vi "OnResize2.vi"(0 "XRef":T20, 1 "Bounds":T18, 2 "Mouse Mods":T16, 3 "State In":T1={"Worker Library Path"=path "", "Block Label"="", "Types"=[], "Selections"=[], "Icon"={"image type"=0, "image depth"=0, "image"=[], "mask"=[], "colors"=[], "Rectangle"={"left"=0, "top"=0, "right"=0, "bottom"=0}}, "Errors"={"Terminals"=[], "Generate"={"status"=FALSE, "code"=0, "source"=""}, "General"={"status"=FALSE, "code"=0, "source"=""}}, "Calculated Sizes"={"Block Width"=0, "Block Height"=0, "Half Width"=0, "Icon Top"=0, "Icon Bottom"=0, "Label Width"=0, "Half Label"=0, "Label Top"=0, "Text Width"=0, "Half Text"=0, "Text Height"=0, "Label Height"=0, "Expanded Width"=0, "Label Bottom"=0, "Expanded Top"=0, "Expanded Bottom"=0, "Expanded Height"=0, "Min Height"=0, "Max Height"=0}, "Special Terminal Indices"={"Action"=-1, "Init"=-1, "Tag"=-1, "State in"=-1, "State out"=-1, "Error"=-1, "Control"=-1}, "Terminals"=[], "First Gen?"=FALSE}) -> (14 "Reply":T14, 15 "Fatal Error Out":T13, 16 "State Out":T1={"Worker Library Path"=path "", "Block Label"="", "Types"=[], "Selections"=[], "Icon"={"image type"=0, "image depth"=0, "image"=[], "mask"=[], "colors"=[], "Rectangle"={"left"=0, "top"=0, "right"=0, "bottom"=0}}, "Errors"={"Terminals"=[], "Generate"={"status"=FALSE, "code"=0, "source"=""}, "General"={"status"=FALSE, "code"=0, "source"=""}}, "Calculated Sizes"={"Block Width"=0, "Block Height"=0, "Half Width"=0, "Icon Top"=0, "Icon Bottom"=0, "Label Width"=0, "Half Label"=0, "Label Top"=0, "Text Width"=0, "Half Text"=0, "Text Height"=0, "Label Height"=0, "Expanded Width"=0, "Label Bottom"=0, "Expanded Top"=0, "Expanded Bottom"=0, "Expanded Height"=0, "Min Height"=0, "Max Height"=0}, "Special Terminal Indices"={"Action"=-1, "Init"=-1, "Tag"=-1, "State in"=-1, "State out"=-1, "Error"=-1, "Control"=-1}, "Terminals"=[], "First Gen?"=FALSE})   [LabVIEW 2022 SP3, in "Flex Block.xnode"]
uses:
  Flex Block.xnode
  <vilib>/XNodeSupport/XNodeXNodeRef.ctl
  <vilib>/XNodeSupport/XNodeRect32.ctl
  <vilib>/XNodeSupport/XNodeInt.ctl
  <vilib>/XNodeSupport/XNodeMouseMods.ctl
  <vilib>/XNodeSupport/XNodeBool.ctl
  State.ctl
  FlexBlocks Support/Type Descriptor.ctl
  FlexBlocks Support/Terminal Direction.ctl
  FlexBlocks Support/Value Mode.ctl
  FlexBlocks Support/Special Terminal.ctl
  <vilib>/picture/picture.llb/imagedata.ctl
  FlexBlocks Support/XNode Errors.ctl
  FlexBlocks Support/Calculated Sizes.ctl
  FlexBlocks Support/Special Terminal Indices.ctl
  FlexBlocks Support/Terminal Status.ctl
  FlexBlocks Support/Terminal State.ctl
  FlexBlocks Support/Terminal Draw Style.ctl
  <vilib>/XNodeSupport/XNodeStringArray.ctl
  <vilib>/XNodeSupport/XNodeString.ctl
  <vilib>/XNodeSupport/XNodeErrorCluster.ctl
  3ea49023-45ad-42f1-9e97-9f20a21117f8.vi
  FlexBlocks Support/_Add Ability Log.vi
  <vilib>/XNodeSupport/NI_XNodeSupport.lvlib
  FlexBlocks Support/FlexBlocks Support.lvlib
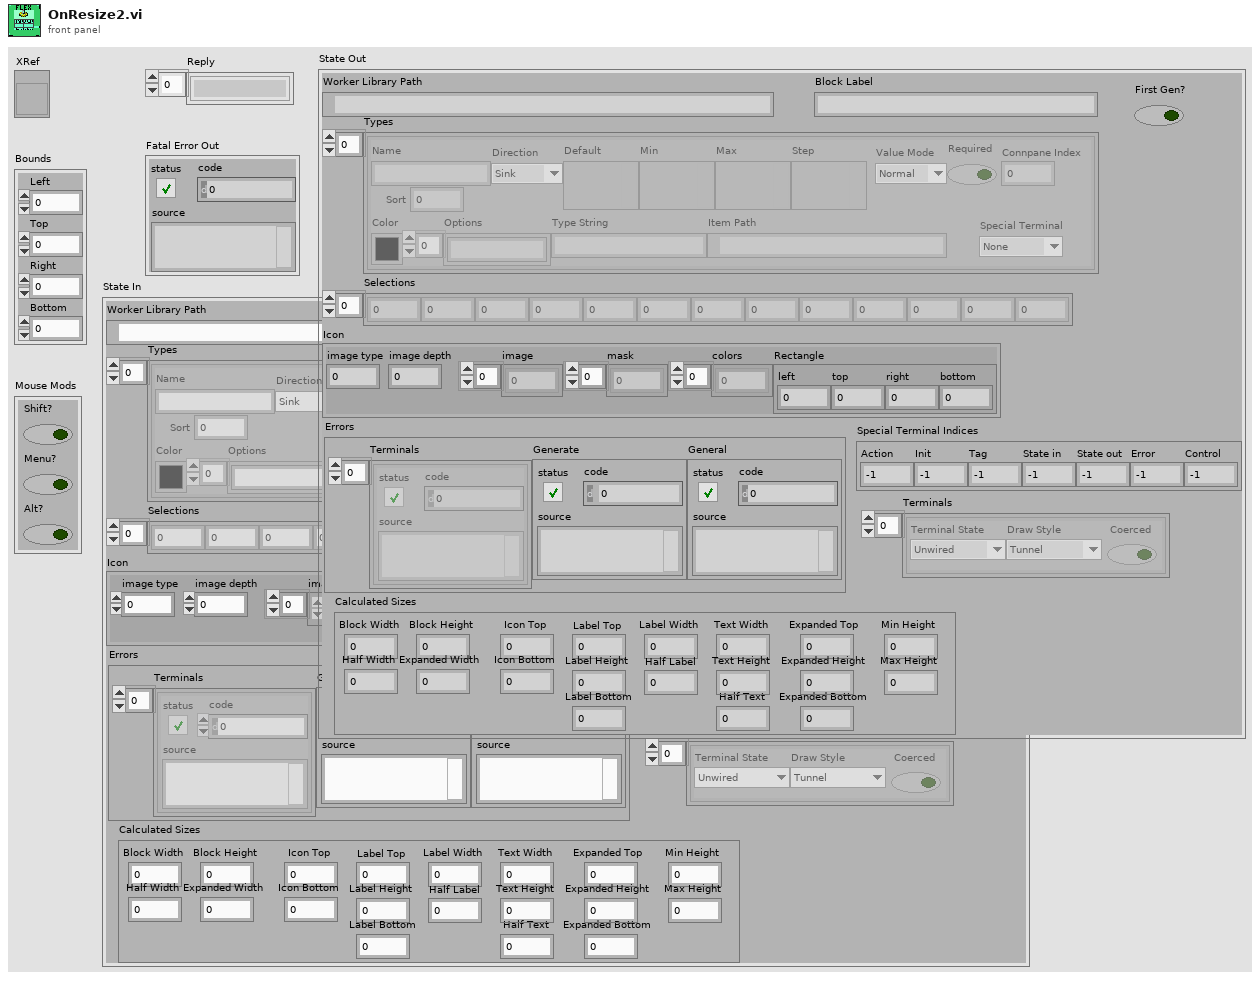
[diagram p1: front panel]
types:
  T1 = typedef "Flex Block.xnode/State.ctl" = cluster{"Worker Library Path":path, "Block Label":string, "Types":T2[], "Selections":i32[], "Icon":T6, "Errors":T7, "Calculated Sizes":T8, "Special Terminal Indices":T9, "Terminals":T10[], "First Gen?":bool}
  T2 = typedef "FlexBlocks Support.lvlib/Type Descriptor.ctl" = cluster{"Name":string, "Direction":T3, "Default":variant, "Min":variant, "Max":variant, "Step":variant, "Value Mode":T4, "Color":u32, "Options":string[], "Type String":string, "Item Path":path, "Required":bool, "Connpane Index":i32, "Special Terminal":T5, "Sort":i32}
  T3 = typedef "FlexBlocks Support.lvlib/Terminal Direction.ctl" = enum16{"Sink", "Source"}
  T4 = typedef "FlexBlocks Support.lvlib/Value Mode.ctl" = enum16{"Normal", "Range", "Select"}
  T5 = typedef "FlexBlocks Support.lvlib/Special Terminal.ctl" = enum16{"None", "Action", "Init", "Tag", "State in", "State out", "Error", "Control"}
  T6 = typedef "imagedata.ctl" = cluster{"image type":i32, "image depth":i32, "image":u8[], "mask":u8[], "colors":u32[], "Rectangle":cluster{"left":i16, "top":i16, "right":i16, "bottom":i16}}
  T7 = typedef "FlexBlocks Support.lvlib/XNode Errors.ctl" = cluster{"Terminals":errorcluster[], "Generate":errorcluster, "General":errorcluster}
  T8 = typedef "FlexBlocks Support.lvlib/Calculated Sizes.ctl" = cluster{"Block Width":i32, "Block Height":i32, "Half Width":i32, "Icon Top":i32, "Icon Bottom":i32, "Label Width":i32, "Half Label":i32, "Label Top":i32, "Text Width":i32, "Half Text":i32, "Text Height":i32, "Label Height":i32, "Expanded Width":i32, "Label Bottom":i32, "Expanded Top":i32, "Expanded Bottom":i32, "Expanded Height":i32, "Min Height":i32, "Max Height":i32}
  T9 = typedef "FlexBlocks Support.lvlib/Special Terminal Indices.ctl" = cluster{"Action":i32, "Init":i32, "Tag":i32, "State in":i32, "State out":i32, "Error":i32, "Control":i32}
  T10 = typedef "FlexBlocks Support.lvlib/Terminal Status.ctl" = cluster{"Terminal State":T11, "Draw Style":T12, "Coerced":bool}
  T11 = typedef "FlexBlocks Support.lvlib/Terminal State.ctl" = enum16{"Unwired", "BadType", "BadRef", "Channel", "Value", "Control Ref"}
  T12 = typedef "FlexBlocks Support.lvlib/Terminal Draw Style.ctl" = enum16{"Tunnel", "BadType", "BadRef", "Channel", "Value", "Control Ref"}
  T13 = typedef "NI_XNodeSupport.lvlib/XNodeErrorCluster.ctl" = errorcluster
  T14 = typedef "NI_XNodeSupport.lvlib/XNodeStringArray.ctl" = T15[]
  T15 = typedef "NI_XNodeSupport.lvlib/XNodeString.ctl" = string
  T16 = typedef "NI_XNodeSupport.lvlib/XNodeMouseMods.ctl" = cluster{"Shift?":T17, "Menu?":T17, "Alt?":T17}
  T17 = typedef "NI_XNodeSupport.lvlib/XNodeBool.ctl" = bool
  T18 = typedef "NI_XNodeSupport.lvlib/XNodeRect32.ctl" = cluster{"Left":T19, "Top":T19, "Right":T19, "Bottom":T19}
  T19 = typedef "NI_XNodeSupport.lvlib/XNodeInt.ctl" = i32
  T20 = typedef "NI_XNodeSupport.lvlib/XNodeXNodeRef.ctl" = refnum<vi>
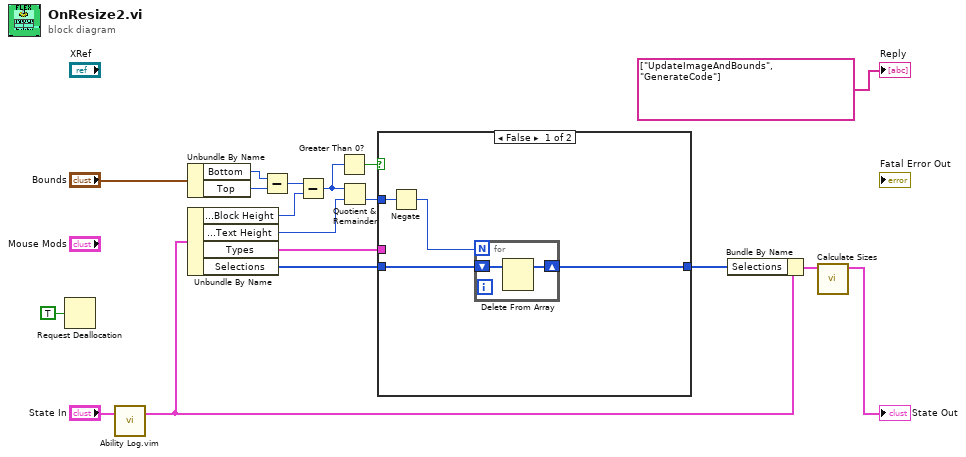
[diagram p0: block diagram]
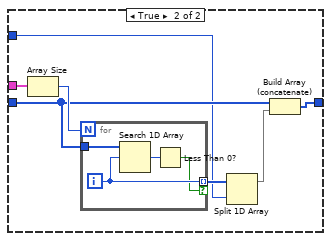
[diagram p2: hidden frame]
diagram:
  n1 = Request Deallocation(TRUE ("flag")) -> ()
  n2 = call "Ability Log.vim"("Wire in"="State In") -> ("Wire out"=w1:T1)  [unwired: 6 in]
  n3 = Unbundle By Name("Bounds") -> ("Bottom"=w15:T19, "Top"=w16:T19)
  n4 = Unbundle By Name(w1) -> ("Calculated Sizes.Block Height"=w13:i32, "Calculated Sizes.Text Height"=w3:i32, "Types"=w12:T2[], "Selections"=w11:i32[])
  n5 = Subtract(x=w15, y=w16) -> (x-y=w14:T19)
  n6 = Subtract(x=w14, y=w13) -> (x-y=w4:T19)
  n7 = Greater Than 0?(x=w4) -> (x > 0?=w8:bool)
  n8 = Quotient & Remainder(x=w4, y=w3) -> (floor(x/y)=w5:T19)  [unwired: 1 out]
  n9 = case shown="False" w8 {
    tunnel: w12 -> [_ w31]
    tunnel: w11 -> [w22 w28]
    tunnel: [w21 w26] -> w10
    tunnel: w5 -> [w20 w25]
    frame False {
      n10 = Negate(x=w20) -> (-x=w19:T19)
      n11 = for {
        N: w19 -> [_]
        shift-right: [w23] -> w21
        shift-left: w22 -> [w24]
        n12 = Delete From Array(array=w24) -> (array with subset deleted=w23:i32[])  [unwired: 2 in, 1 out]
      }
    }
    frame True {
      n13 = Array Size(array=w31) -> (size(s)=w30:i32)
      n14 = for {
        N: w30 -> [_]
        tunnel: w28 -> [w35]
        tunnel: [w33] -> w29 mode=indexing if=w32
        i -> [w33]
        n15 = Search 1D Array(1D array=w35, element=w33) -> (index of element=w34:i32)  [unwired: 1 in]
        n16 = Less Than 0?(x=w34) -> (x < 0?=w32:bool)
      }
      n17 = Split 1D Array(array=w29, index=w25) -> (first subarray=w27:i32[])  [unwired: 1 out]
      n18 = Build Array (concatenate)(w28, w27) -> (w26:i32[])
    }
  }
  n19 = Bundle By Name(cluster=w1, "Selections"=w10) -> (w7:T1)
  n20 = call "Calculate Sizes.vi"("State In"=w7) -> ("State"=→"State Out":T1)  [unwired: 10 in]
  "Reply" <- T14 ["UpdateImageAndBounds", "GenerateCode"] ("Reply")
